vi "ConfirmFile.vi"(2 "Error In":errorcluster, 3 "Filename IN":string, 4 "Pathname IN":string) -> (0 "Error Out":errorcluster, 1 "Filename:":string)   [LabVIEW 2013]
uses:
  globals/QC_RunInformation.vi
panel:
  out "Pathname":string
  out "Folder already existed":bool
  in  "stop":bool
  # "Saving Data File"
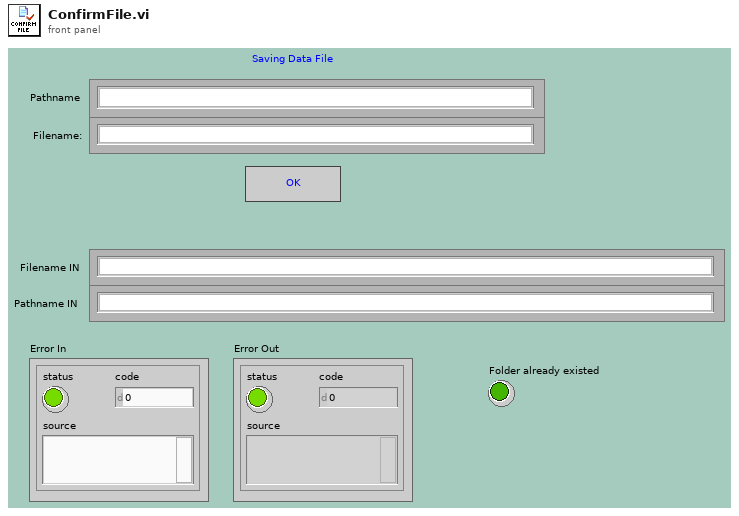
[diagram p1: front panel]
types:
  T1 = cluster{"Sensor Serial No.:":string, "Wafer Serial No.:":string, "Batch:":string, "Manufacturer:":string, "Device Category:":string, "Database Serial No.:":string, "Initiated:":string, "Test":string, "Instruments used:":string, "Probeplan used:":string, "End of Run comment:":string, "User:":string}
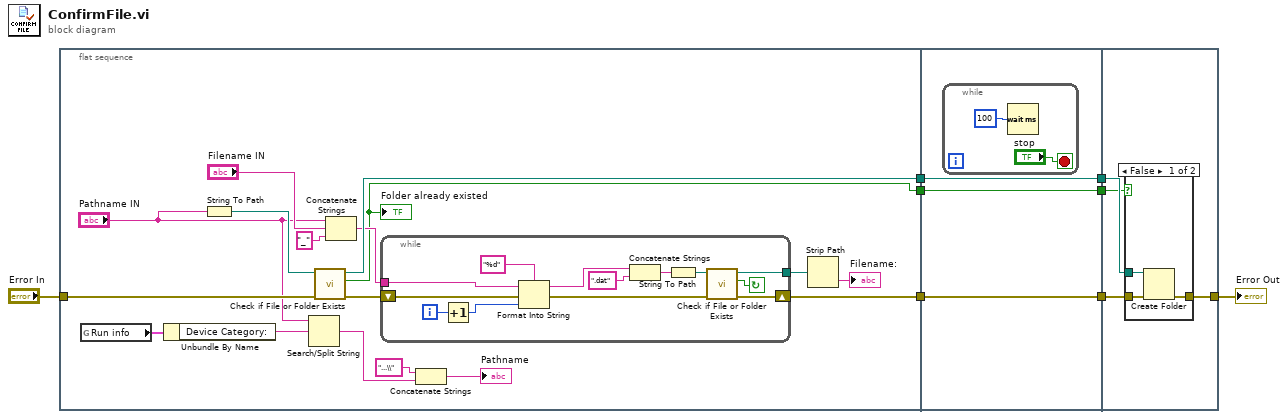
[diagram p0: block diagram]
diagram:
  n1 = flat-sequence {
    tunnel: "Error In" -> [w25]
    tunnel: [w20] -> w5
    tunnel: [w23] -> w4
    tunnel: [w18] -> w2
    tunnel: [w41] -> w6
    tunnel: w5 -> [w41]
    tunnel: w4 -> [w40]
    tunnel: [w40] -> w3
    tunnel: w2 -> [w39]
    tunnel: [w39] -> w1
    tunnel: [w47] -> w7
    tunnel: w6 -> [w46]
    tunnel: w3 -> [w45]
    tunnel: w1 -> [w44]
    frame #0 {
      n2 = global read "QC_RunInformation.vi" "Run info"() -> (w13:T1)
      n3 = Unbundle By Name(w13) -> ("Device Category:"=w12:string)
      n4 = String To Path(string="Pathname IN") -> (path=w24:path)
      n5 = Search/Split String(string="Pathname IN", search string/char (-)=w12) -> (match + rest of string=w10:string)  [unwired: 1 in, 2 out]
      n6 = call <vilib>:"Check if File or Folder Exists.vi"("error in (no error)"=w25, "path"=w24) -> ("error out"=w21:errorcluster, "file or folder exists?"=w18:bool, "dup path"=w23:path)  [unwired: 7 in]
      "Folder already existed" <- w18
      n7 = Concatenate Strings("Pathname IN", "Filename IN", "_") -> (w19:string)
      n8 = while {
        shift-right: [w37] -> w20
        shift-left: w21 -> [w31]
        tunnel: w19 -> [w35]
        tunnel: [w29] -> w16
        i -> [w36]
        stop <- w38 continue-if-true
        n9 = Increment(x=w36) -> (x+1=w33:i32)
        n10 = Format Into String(format string="%d", initial string=w35, error in=w31, w33) -> (resulting string=w28:string, error out=w30:errorcluster)
        n11 = Concatenate Strings(w28, ".dat") -> (w26:string)
        n12 = String To Path(string=w26) -> (path=w32:path)
        n13 = call <vilib>:"Check if File or Folder Exists.vi"("error in (no error)"=w30, "path"=w32) -> ("error out"=w37:errorcluster, "file or folder exists?"=w38:bool, "dup path"=w29:path)  [unwired: 7 in]
      }
      n14 = Concatenate Strings("...\\", w10) -> (→"Pathname":string)
      n15 = Strip Path(path=w16) -> (name=→"Filename:":string)  [unwired: 1 out]
    }
    frame #1 {
      n16 = while {
        stop <- "stop" stop-if-true
        n17 = Wait (ms)(milliseconds to wait=u32 100) -> ()  [unwired: 1 out]
      }
    }
    frame #2 {
      n18 = case shown="False" w44 {
        tunnel: w46 -> [w50 w51]
        tunnel: w45 -> [w49 _]
        tunnel: [w48 w51] -> w47
        frame False {
          n19 = Create Folder(path (use dialog)=w49, error in=w50) -> (error out=w48:errorcluster)  [unwired: 1 in, 2 out]
        }
        frame True {
        }
      }
    }
  }
  "Error Out" <- w7
